vi "Actor Core.vi"(8 "error in":errorcluster, 11 "WS Test Server in":refnum<class "WS Test Server.lvclass">) -> (0 "error out":errorcluster, 3 "Actor out":refnum<class "Actor.lvclass">)   [LabVIEW 2016, in "Test Server Manager.lvlib" / "WS Test Server.lvclass"]
doc: "(<B>Filename</B>: Actor Framework.lvlib:Actor.lvclass:Actor Core.vi)\n\nReceives messages to the actor, reacts to them, and initiates any error handling that may shut the actor down.\n\nDescendant classes may override this VI to append parallel tasks for the actor to complete while it handles messages. Overrides use the Call Parent Method node."
uses:
  WS Test Server.lvclass
  C:/Program Files (x86)/National Instruments/LabVIEW 2016/vi.lib/ActorFramework/Actor/Actor.lvclass
  <vilib>/ActorFramework/Actor/Actor.lvclass
  WebSocket Actor/WebSocket Server/typedefs/Listener Settings.ctl
  WS Test Server Messages/WebSocket Server Enqueuer Msg/WebSocket Server Enqueuer Msg.lvclass
  C:/Projects/Shared Libraries/WebSocket Actor/WebSocket Actor/Abstract Messages/WebSocket Server-Service Enqueuer Msg/WebSocket Server-Service Enqueuer Msg.lvclass
  <vilib>/ActorFramework/Actor/Actor.lvclass/Actor.ctl
  <vilib>/ActorFramework/Message Enqueuer/Message Enqueuer.lvclass/Message Enqueuer.ctl
  WS Test Server.lvclass/WS Test Server.ctl
  <vilib>/ActorFramework/Message Enqueuer/Init from Existing Queue.vi
  <vilib>/MGI/Monitored Actor/Monitored Actor/Monitored Actor/Monitored Actor.lvclass
  <vilib>/ActorFramework/Message Enqueuer/Message Enqueuer.lvclass
  WebSocket Actor/WebSocket Server Manager Messages/Launch Server Msg/Launch Server Msg.lvclass
  WebSocket Actor/WebSocket Server/WebSocket Server.lvclass
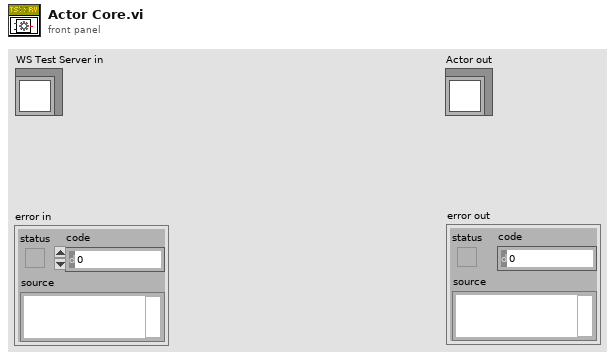
[diagram p1: front panel]
types:
  T1 = typedef "WebSocket Actors.lvlib/WebSocket Server.lvclass/Listener Settings.ctl" = cluster{"resolve remote address (T)":bool, "timeout ms (-1)":i32, "net address":u32, "port":u16}
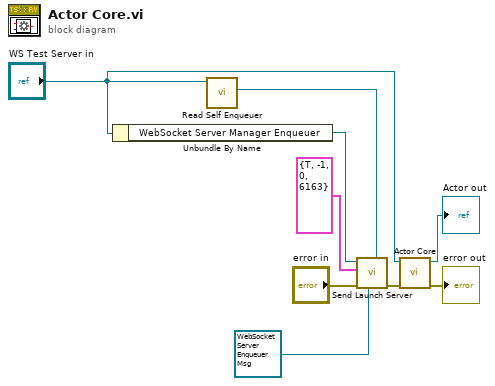
[diagram p0: block diagram]
diagram:
  n1 = Unbundle By Name("WS Test Server in") -> ("WebSocket Server Manager Enqueuer"=w2:refnum<class "Message Enqueuer.lvclass">)
  n2 = call <vilib>:"Read Self Enqueuer.vi"("Actor"="WS Test Server in") -> ("Self Enqueuer"=w4:refnum<class "Message Enqueuer.lvclass">)  [unwired: 10 in]
  n3 = call "Send Launch Server.vi"("Client Enqueuer"=w4, "Receive Server Enqueuer Handler"=refnum<class "WebSocket Server Enqueuer Msg.lvclass"> refnum ("Echo Broadcast Test With Server Manager.lvlib:WebSocket Server Enqueuer Msg.lvclass"), "error in (no error)"="error in", "Listener Settings"=T1 {"resolve remote address (T)"=TRUE, "timeout ms (-1)"=-1, "net address"=0, "port"=6163}, "Message Enqueuer in"=w2) -> ("error out"=w5:errorcluster)  [unwired: 5 in, 1 out]
  n4 = call-parent "Actor Core.vi"("error in"=w5, "Actor in"="WS Test Server in") -> ("error out"=→"error out":errorcluster, "Actor out"=→"Actor out":refnum<class "Actor.lvclass">)  [unwired: 8 in]
